vi "Which_Trav_Setup.vi"(0 "Extra Command String":string) -> (1 "Index":i32, 2 "Traverse Setups":string[](array[string]), 3 "XYZ Offset of 2nd Traverse":sgl[](array[numeric]))   [LabVIEW 2018]
uses:
  Globals/Extra_Commands_Global.vi
  Globals/Trav_pos_global.vi
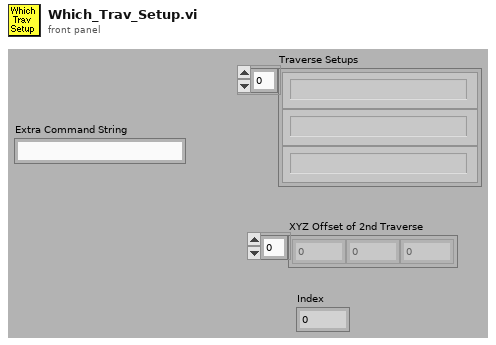
[diagram p1: front panel]
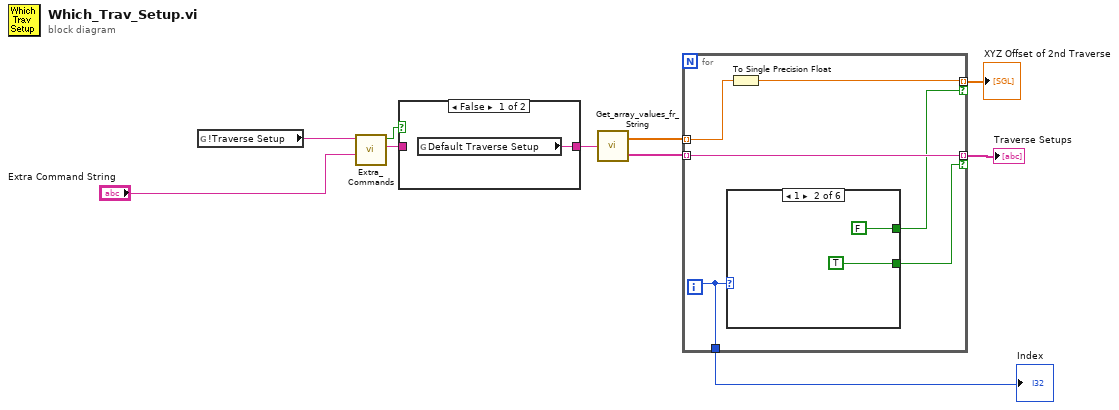
[diagram p0: block diagram]
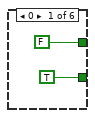
[diagram p2: hidden frame]
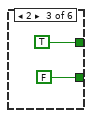
[diagram p3: hidden frame]
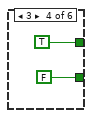
[diagram p4: hidden frame]
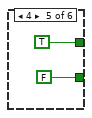
[diagram p5: hidden frame]
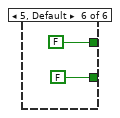
[diagram p6: hidden frame]
diagram:
  n1 = global read "Extra_Commands_Global.vi" "!Traverse Setup"() -> (w8:string)
  n2 = call "Extra_Commands.vi"("String to Search"="Extra Command String", "Command"=w8) -> ("String Value"=w10:string, "Command Found"=w9:bool)  [unwired: 1 in, 3 out]
  n3 = case shown="False" w9 {
    tunnel: [w11 w12] -> w6
    tunnel: w10 -> [_ w12]
    frame False {
      n4 = global read "Trav_pos_global.vi" "Default Traverse Setup"() -> (w11:string)
    }
    frame True {
    }
  }
  n5 = call "Get_array_values_fr_String.vi"("String Value"=w6) -> ("Numeric Array"=w4:dbl[], "String array"=w5:string[])
  n6 = for {
    tunnel: w5 -> [w18] mode=indexing
    tunnel: [w18] -> w2 mode=indexing if=w17
    tunnel: [w14] -> w3 mode=indexing if=w15
    tunnel: w4 -> [w16] mode=indexing
    tunnel: [w13] -> w1
    i -> [w13]
    n7 = case shown="1" w13 {
      tunnel: [TRUE TRUE FALSE FALSE FALSE FALSE] -> w17
      tunnel: [FALSE FALSE TRUE TRUE TRUE FALSE] -> w15
      frame 0 {
      }
      frame 1 {
      }
      frame 2 {
      }
      frame 3 {
      }
      frame 4 {
      }
      frame 5, Default {
      }
    }
    n8 = To Single Precision Float(number=w16) -> (single precision float=w14:sgl)
  }
  "Traverse Setups" <- w2
  "XYZ Offset of 2nd Traverse" <- w3
  "Index" <- w1
